vi "YKMW100 Scale 4_20 to Percent.vi"(8 "error in (no error)":errorcluster, 10 "Previous Data":dbl, 11 "mA":dbl) -> (0 "error out":errorcluster, 3 "Valve (% Open)":dbl)   [LabVIEW 2023]
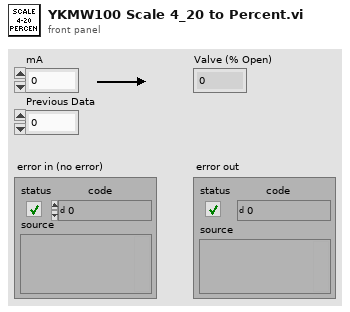
[diagram p1: front panel]
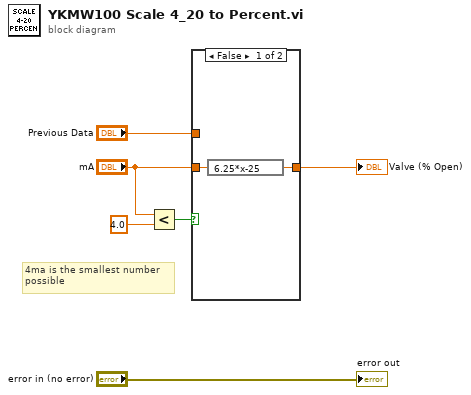
[diagram p0: block diagram]
diagram:
  # "4ma is the smallest number \npossible"
  n1 = Less?(x="mA", y=4.0) -> (x < y?=w5:bool)
  n2 = case shown="False" w5 {
    tunnel: [w8 w9] -> w6
    tunnel: "mA" -> [w7 _]
    tunnel: "Previous Data" -> [_ w9]
    frame False {
      n3 = expression code="6.25*x-25"(w7) -> (w8:dbl)
    }
    frame True {
    }
  }
  "Valve (% Open)" <- w6
  "error out" <- "error in (no error)"
